vi "hexToNum_LE.vi"(1 "String":string) -> (0 "Numeric":dbl)   [LabVIEW 2015]
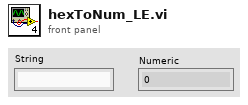
[diagram p1: front panel]
types:
  T1 = enum16{"big-endian, network order", "native, host order", "little-endian"}
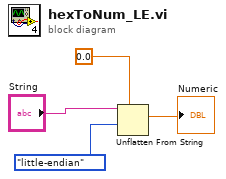
[diagram p0: block diagram]
diagram:
  n1 = Unflatten From String(type=sgl 0.0, binary string="String", byte order (0:big-endian, network order)=T1."little-endian") -> (value=→"Numeric":sgl)  [unwired: 2 in, 2 out]
